vi "Pixel Width.vi"(9 "Pixels per Char":i32=8, 10 "Array":string[](array[string])) -> (1 "Widths":i32[](array[numeric]), 2 "Pixel Width":i32)   [LabVIEW 2013]
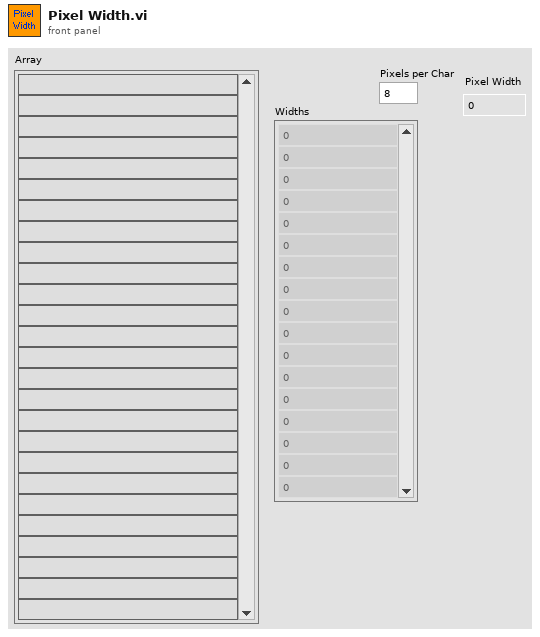
[diagram p1: front panel]
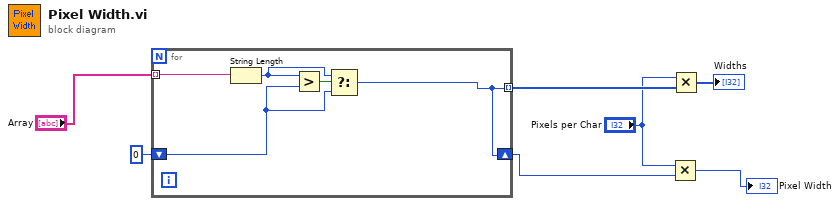
[diagram p0: block diagram]
diagram:
  n1 = for {
    shift-right: [w8] -> w5
    shift-left: 0 -> [w9]
    tunnel: "Array" -> [w10] mode=indexing
    tunnel: [w8] -> w3 mode=indexing
    n2 = String Length(string=w10) -> (length=w12:i32)
    n3 = Greater?(x=w12, y=w9) -> (0:w11:bool)
    n4 = Select(t=w12, s=w11, f=w9) -> (s? t:f=w8:i32)
  }
  n5 = Multiply(x="Pixels per Char", y=w5) -> (x*y=→"Pixel Width":i32)
  n6 = Multiply(x="Pixels per Char", y=w3) -> (x*y=→"Widths":i32[])
